vi "Write q ref.vi"(8 "error in (no error)":errorcluster, 10 "q ref":refnum<vi>, 11 "Analyze Results q-Factor in":refnum<class "Analyze Results q-Factor.lvclass">) -> (0 "error out":errorcluster, 3 "Analyze Results q-Factor out":refnum<class "Analyze Results q-Factor.lvclass">)   [LabVIEW 2014, in "Analyze Results q-Factor.lvclass"]
uses:
  Analyze Results q-Factor.lvclass
  Analyze Results q-Factor.lvclass/Analyze Results q-Factor.ctl
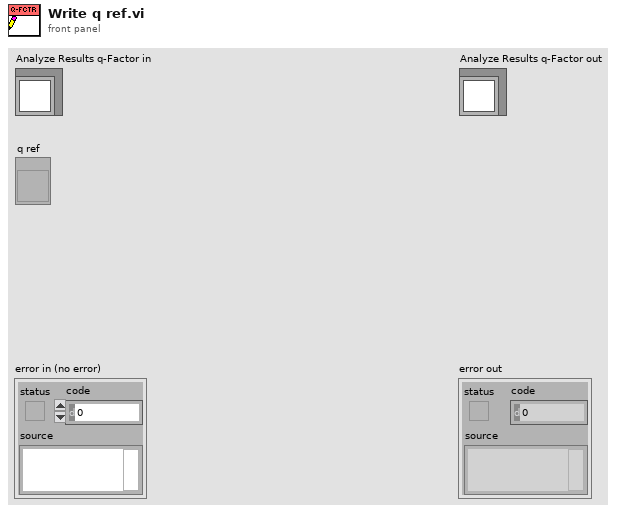
[diagram p1: front panel]
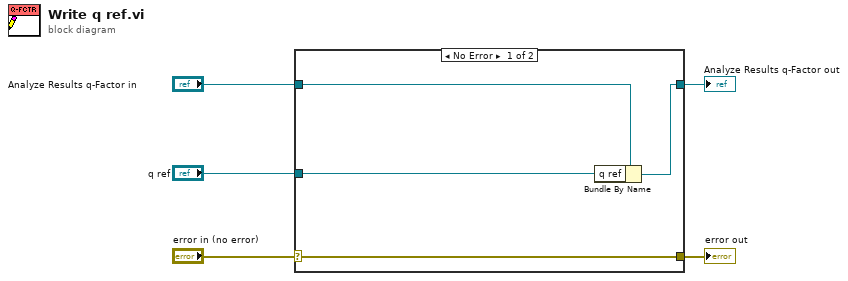
[diagram p0: block diagram]
diagram:
  n1 = case shown="No Error" "error in (no error)" {
    selector: "error in (no error)" -> [w9 w10]
    tunnel: [w9 w10] -> w4
    tunnel: [w7 w11] -> w2
    tunnel: "Analyze Results q-Factor in" -> [w8 w11]
    tunnel: "q ref" -> [w6 _]
    frame No Error {
      n2 = Bundle By Name(cluster=w8, "q ref"=w6) -> (w7:refnum<class "Analyze Results q-Factor.lvclass">)
    }
    frame Error {
    }
  }
  "error out" <- w4
  "Analyze Results q-Factor out" <- w2
